vi "Text File Reader.vi"(1 "file (use dialog)":path=path "C:/Users/developer/Desktop/Auton1.txt") -> ()   [LabVIEW 2012]
panel:
  out "Power":i32
  out "Direction":i32
  out "Array":T1(array[cluster])
  out "Text Information":string
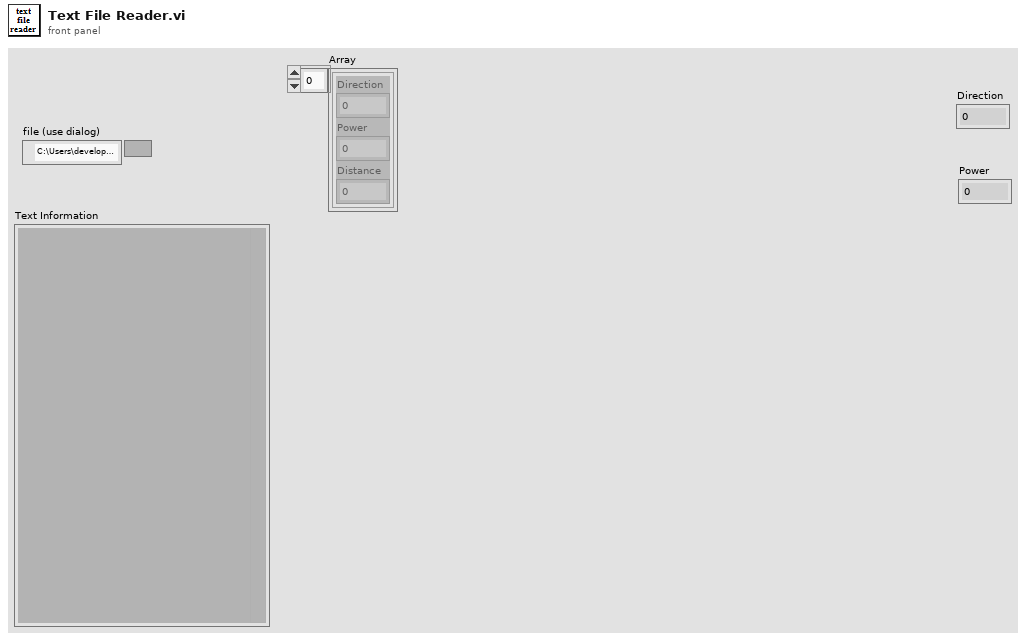
[diagram p1: front panel]
types:
  T1 = cluster{"Direction":i32, "Distance":i32, "Power":i32}[]
  T2 = cluster{"Direction":i32, "Distance":i32, "Power":i32}
  T3 = cluster{"[0]":i32, "[1]":i32, "[2]":i32, "[3]":i32, "[4]":i32, "[5]":i32, "[6]":i32, "[7]":i32, "[8]":i32}
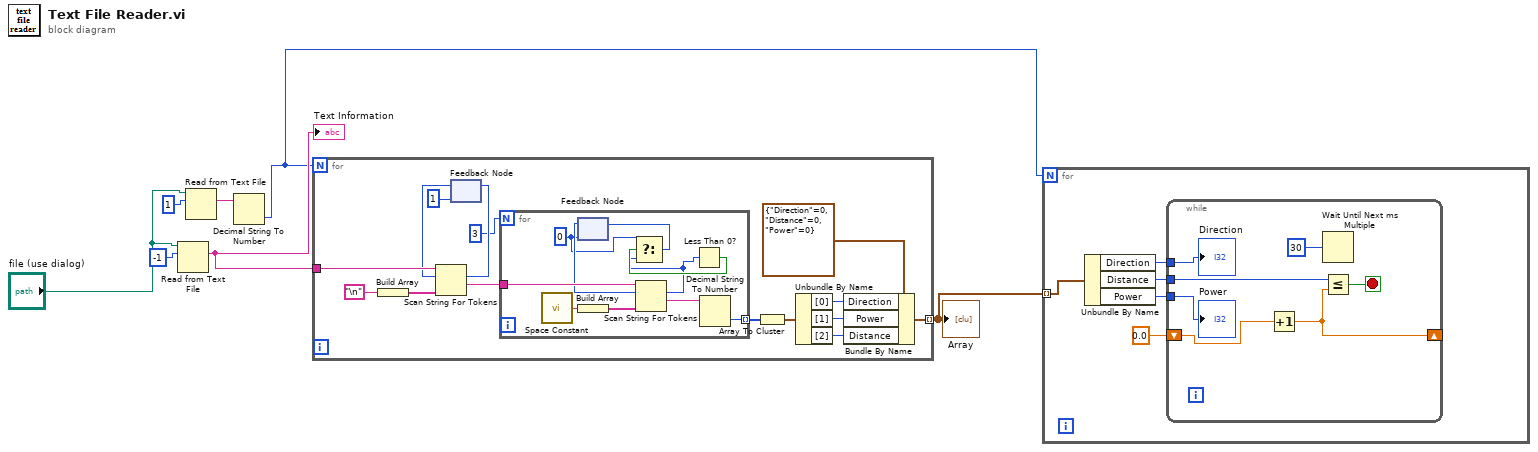
[diagram p0: block diagram]
diagram:
  n1 = Read from Text File(file (use dialog)="file (use dialog)", count=-1) -> (text=w6:string)  [unwired: 1 in, 4 out]
  "Text Information" <- w6
  n2 = Read from Text File(file (use dialog)="file (use dialog)", count=1) -> (text=w3:string)  [unwired: 1 in, 4 out]
  n3 = Decimal String To Number(string=w3) -> (number=w2:i32)  [unwired: 2 in, 1 out]
  n4 = for {
    N: w2 -> [_]
    tunnel: w6 -> [w22]
    tunnel: [w8] -> w1 mode=indexing
    n5 = Build Array("\n") -> (w19:string[])
    n6 = feedback #1(1) -> (w20:i32)
    n7 = Scan String For Tokens(6:w19, 8:w20, 9:w22) -> (1:w18:string, 2:w21:i32)  [unwired: 3 in, 2 out]
    n8 = feedback-in #1(w21) -> ()
    n9 = for {
      N: 3 -> [_]
      tunnel: w18 -> [w32]
      tunnel: [w27] -> w14 mode=indexing
      w25 = 0 ("offset past token")
      n10 = call <vilib>:"Space Constant.vi"() -> ("String"=w30:string)
      n11 = feedback #2(w25) -> (w31:i32)
      n12 = Build Array(w30) -> (w29:string[])
      n13 = Scan String For Tokens(6:w29, 8:w31, 9:w32) -> (1:w28:string, 2:w23:i32)  [unwired: 3 in, 2 out]
      n14 = Less Than 0?(x=w23) -> (x < 0?=w26:bool)
      n15 = Select(t=w25, s=w26, f=w23) -> (s? t:f=w24:i32)
      n16 = feedback-in #2(w24) -> ()
      n17 = Decimal String To Number(string=w28) -> (number=w27:i32)  [unwired: 2 in, 1 out]
    }
    n18 = Array To Cluster(array=w14) -> (cluster=w13:T3)
    n19 = Unbundle By Name(w13) -> ("[0]"=w12:i32, "[1]"=w11:i32, "[2]"=w10:i32)
    n20 = Bundle By Name(cluster=T2 {"Direction"=0, "Distance"=0, "Power"=0} ("input cluster"), "Direction"=w12, "Power"=w11, "Distance"=w10) -> (w8:T2)
  }
  "Array" <- w1
  n21 = for {
    N: w2 -> [_]
    tunnel: w1 -> [w37] mode=indexing
    n22 = Unbundle By Name(w37) -> ("Direction"=w34:i32, "Distance"=w36:i32, "Power"=w35:i32)
    n23 = while {
      tunnel: w36 -> [w43]
      tunnel: w35 -> [w42]
      tunnel: w34 -> [w41]
      shift-right: [w38] -> _
      shift-left: 0.0 -> [w39]
      stop <- w44 stop-if-true
      n24 = Increment(x=w39) -> (x+1=w38:dbl)
      n25 = Wait Until Next ms Multiple(millisecond multiple=u32 30) -> ()  [unwired: 1 out]
      n26 = Less Or Equal?(x=w43, y=w38) -> (x <= y?=w44:bool)
      "Direction" <- w41
      "Power" <- w42
    }
  }
